vi "Match (String).vi"(8 "error in (no error)":errorcluster, 9 "Base URL String (Empty)":string, 10 "URL String":string, 11 "URLPattern in":refnum<class "URLPattern.lvclass">) -> (0 "error out":errorcluster, 1 "Matches?":bool, 2 "Result":refnum<class "URLPatternResult.lvclass">, 3 "URLPattern out":refnum<class "URLPattern.lvclass">)   [LabVIEW 2020, in "Stream.lvlib" / "URLPattern.lvclass"]
uses:
  URLPattern.lvclass
  URLPatternResult/URLPatternResult.lvclass
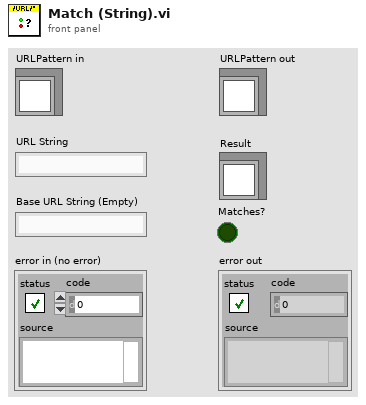
[diagram p1: front panel]
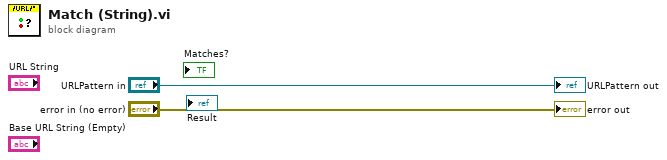
[diagram p0: block diagram]
diagram:
  "error out" <- "error in (no error)"
  "URLPattern out" <- "URLPattern in"
